vi "_Object Tester.vi"() -> ()   [LabVIEW 2025, in "USB IO.lvlib" / "USB IO.lvclass"]
uses:
  USB IO generic/USB IO.lvclass
  USB IO generic/USB IO.lvclass/USB IO.ctl
  <vilib>/Handler Framework/Handler Framework.lvlib
  Hardware Selection.ctl
  USB-6000/USB-6000.lvclass
  <vilib>/Handler Framework/CmdQueue/Enqueue Single.vi
  Arduino Uno/Arduino Uno.lvclass
  C:/Users/grove/Desktop/LabVIEW/Git/dqmh-lvoop-template/Libraries/USB IO/Classes/USB IO generic/USB IO.lvclass
  C:/Users/grove/Desktop/LabVIEW/Git/dqmh-lvoop-template/Libraries/USB IO/Classes/USB-6000/USB-6000.lvclass
  C:/Users/grove/Desktop/LabVIEW/Git/dqmh-lvoop-template/Libraries/USB IO/Classes/Arduino Uno/Arduino Uno.lvclass
panel:
  in  "stop":bool
  out "Waveform Chart":dbl[](graph)
  out "Array":dbl[](array[numeric])
  out "error out 2":errorcluster
  out "error out":errorcluster
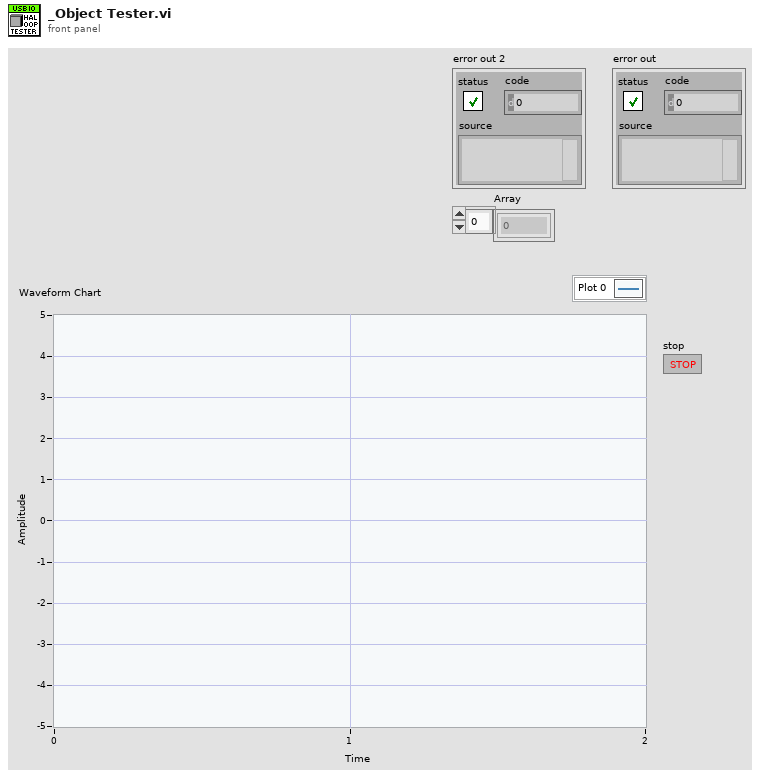
[diagram p1: front panel]
types:
  T1 = typedef "Hardware Selection.ctl" = enum16{"Simulation", "USB-6000", "USB-6001", "Arduino Uno"}
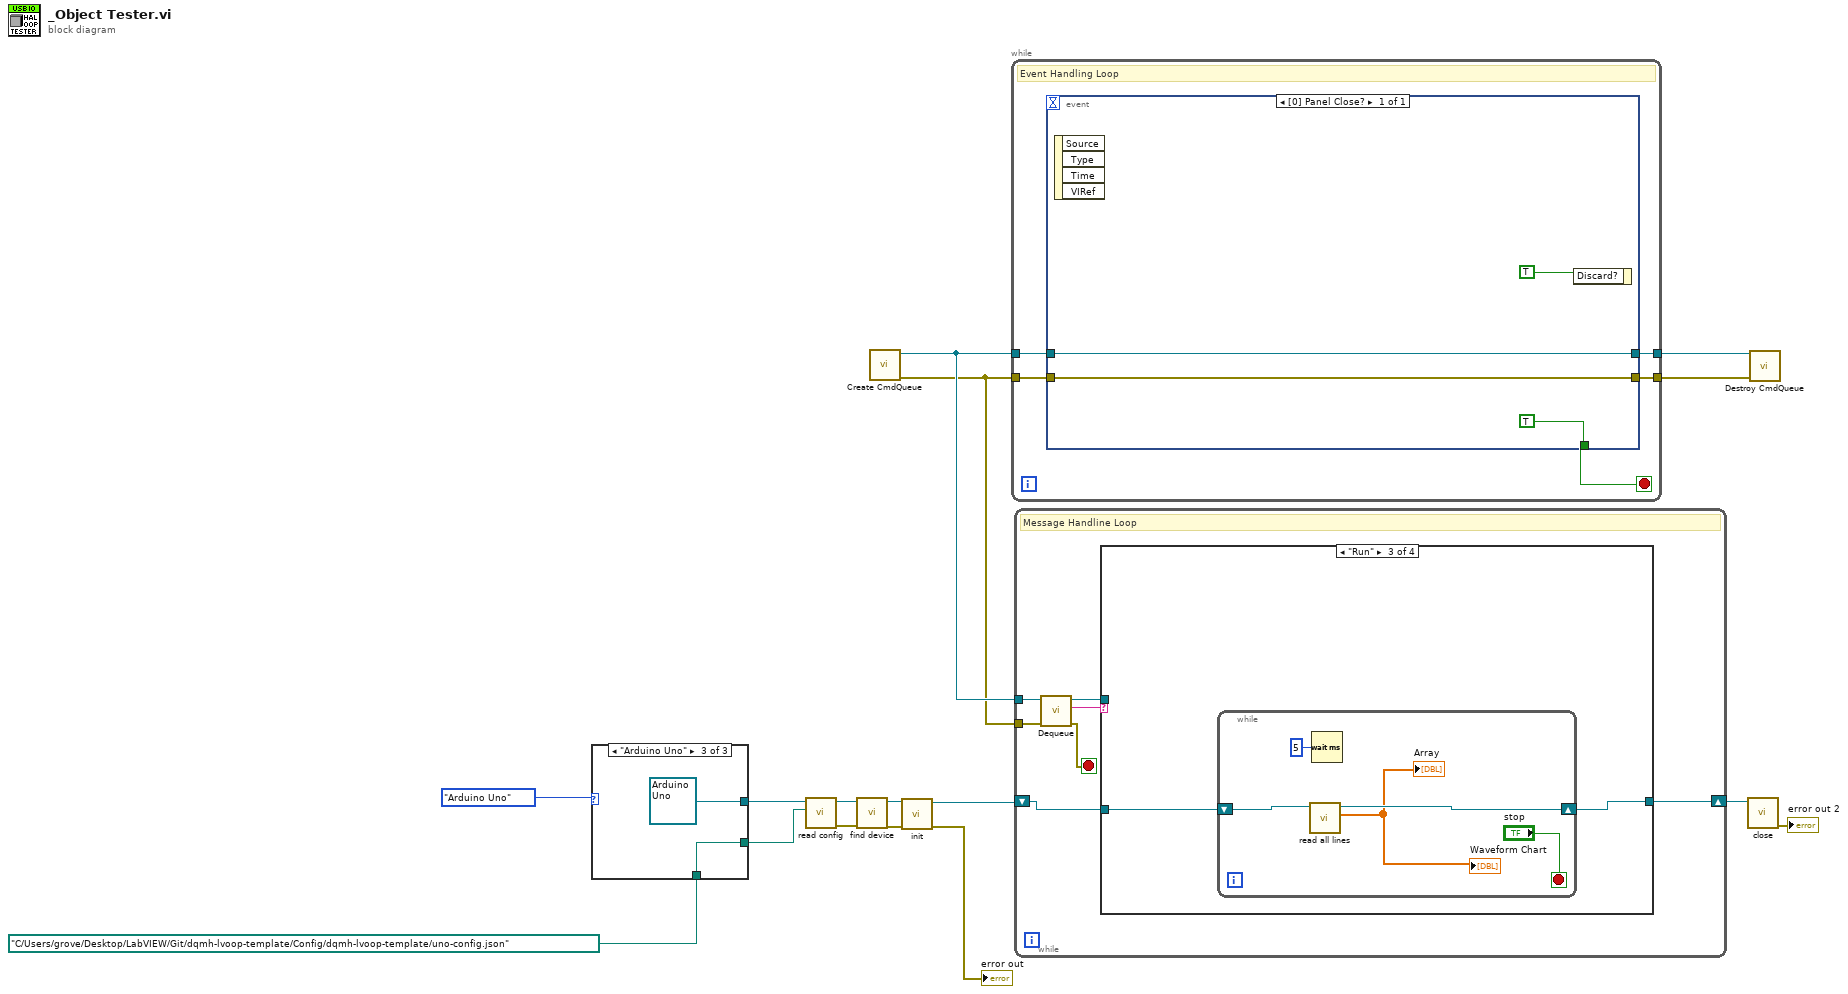
[diagram p0: block diagram]
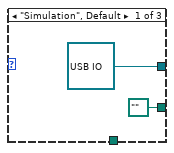
[diagram p2: hidden frame]
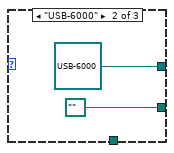
[diagram p3: hidden frame]
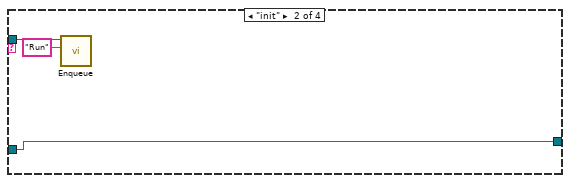
[diagram p5: hidden frame]
diagram:
  n1 = case shown="\"Arduino Uno\"" Hardware_Selection."Arduino Uno" {
    tunnel: [refnum<class "USB IO.lvclass"> refnum ("USB IO.lvlib:USB IO.lvclass") refnum<class "USB-6000.lvclass"> refnum ("USB IO.lvlib:USB-6000.lvclass") refnum<class "Arduino Uno.lvclass"> refnum ("USB IO.lvlib:Arduino Uno.lvclass")] -> w3
    tunnel: [path "" ("Path") path "" ("Path") w21] -> w2
    tunnel: path "C:/Users/grove/Desktop/LabVIEW/Git/dqmh-lvoop-template/Config/dqmh-lvoop-template/uno-config.json" ("Path") -> [_ _ w21]
    frame "Simulation", Default {
    }
    frame "USB-6000" {
    }
    frame "Arduino Uno" {
    }
  }
  n2 = call-dynamic "read config.vi"("Path"=w2, "USB IO in"=w3) -> ("error out"=w4:errorcluster, "USB IO out"=w5:refnum<class "USB IO.lvclass">)  [unwired: 8 in]
  n3 = call-dynamic "find device.vi"("error in (no error)"=w4, "USB IO in"=w5) -> ("error out"=w9:errorcluster, "USB IO out"=w10:refnum<class "USB IO.lvclass">)  [unwired: 8 in]
  n4 = call <vilib>:"Create CmdQueue.vi"() -> ("error out"=w15:errorcluster, "CmdQueue out"=w16:refnum<queue>)  [unwired: 10 in]
  n5 = call-dynamic "init.vi"("error in (no error)"=w9, "USB IO in"=w10) -> ("error out"=→"error out":errorcluster, "USB IO out"=w8:refnum<class "USB IO.lvclass">)  [unwired: 8 in]
  n6 = while {
    tunnel: w16 -> [w26]
    tunnel: w15 -> [w25]
    tunnel: [w24] -> w14
    tunnel: [w23] -> w13
    stop <- w27 stop-if-true
    # "Event Handling Loop"
    n7 = event shown="[0] Panel Close?" {
      selector: _ -> [_]
      dyn-events: _ -> [_]
      timeout: _ -> [_]
      tunnel: [TRUE] -> w27
      tunnel: w26 -> [w29]
      tunnel: w25 -> [w28]
      tunnel: [w29] -> w24
      tunnel: [w28] -> w23
      event Panel Close? {
        n8 = event-data() -> ()  [unwired: 1 in, 4 out]
        n9 = event-data("Discard?"=TRUE) -> ()  [unwired: 1 in, 1 out]
      }
    }
  }
  n10 = while {
    tunnel: w16 -> [w38]
    tunnel: w15 -> [w37]
    shift-right: [w32] -> w11
    shift-left: w8 -> [w33]
    stop <- w36 stop-if-true
    # "Message Handline Loop"
    n11 = call <vilib>:"Dequeue.vi"("error in (no error)"=w37, "CmdQueue in"=w38) -> ("error out"=w36:errorcluster, "cmd"=w35:string, "CmdQueue out"=w34:refnum<queue>)  [unwired: 5 in, 2 out]
    n12 = case shown="\"Run\"" w35 {
      tunnel: w34 -> [_ w42 _ _]
      tunnel: w33 -> [w39 w40 w44 w50]
      tunnel: [w39 w40 w43 w50] -> w32
      frame Default {
      }
      frame "init" {
        n13 = call-poly <vilib>:"Enqueue.vi"("Command"="Run", "CmdQueue in"=w42) -> ()  [unwired: 8 in, 2 out]
      }
      frame "Run" {
        n14 = while {
          shift-right: [w48] -> w43
          shift-left: w44 -> [w49]
          stop <- "stop" stop-if-true
          n15 = call-dynamic "read all lines.vi"("USB IO in"=w49) -> ("Array"=→"Array" →"Waveform Chart":dbl[], "USB IO out"=w48:refnum<class "USB IO.lvclass">)  [unwired: 8 in, 1 out]
          n16 = Wait (ms)(milliseconds to wait=u32 5) -> ()  [unwired: 1 out]
        }
      }
      frame "shutdown" {
      }
    }
  }
  n17 = call-dynamic "close.vi"("USB IO in"=w11) -> ("error out"=→"error out 2":errorcluster)  [unwired: 9 in, 1 out]
  n18 = call <vilib>:"Destroy CmdQueue.vi"("error in (no error)"=w13, "CmdQueue in"=w14) -> ()  [unwired: 9 in, 1 out]
